vi "Action.vi"(7 "Assert Message":T1, 8 "error in (no error)":errorcluster, 11 "Fail Action Base in":refnum<class "Fail Action Base.lvclass">) -> (0 "error out":errorcluster)   [LabVIEW 2016, in "Assert API Components.lvlib" / "Log Assert Core.lvlib" / "Fail Action Base.lvclass"]
doc: "Dynamic dispatch vi which is triggered when an assert fails and the failure action is set to None. Does nothing"
uses:
  Fail Action Base.lvclass
  Message Data.ctl
  Failure Actions.ctl
  Assert API Components.lvlib
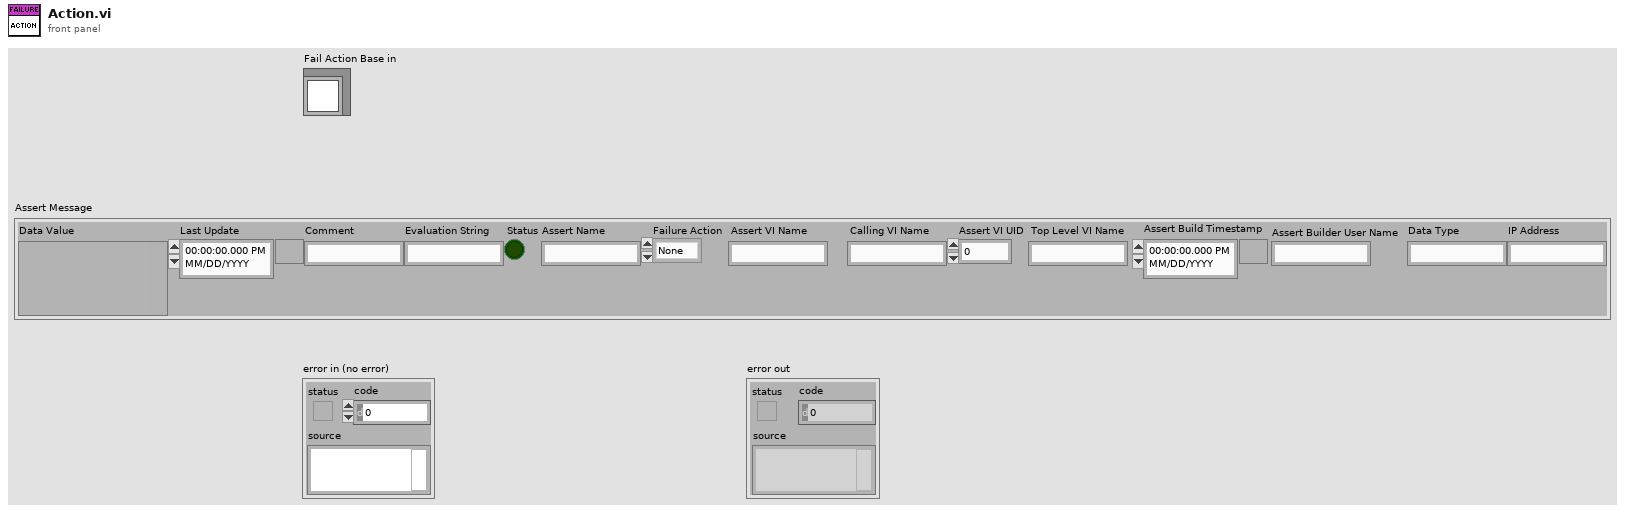
[diagram p1: front panel]
types:
  T1 = typedef "Assert API Components.lvlib/Message Data.ctl" = cluster{"Data Value":variant, "Last Update":timestamp, "Comment":string, "Evaluation String":string, "Status":bool, "Assert Name":string, "Failure Action":T2, "Assert VI Name":string, "Calling VI Name":string, "Assert VI UID":i32, "Top Level VI Name":string, "Assert Build Timestamp":timestamp, "Assert Builder User Name":string, "Data Type":string, "IP Address":string}
  T2 = typedef "Assert API Components.lvlib/Failure Actions.ctl" = enum16{"None", "Log To File", "Pause Execution", "Abort Execution"}
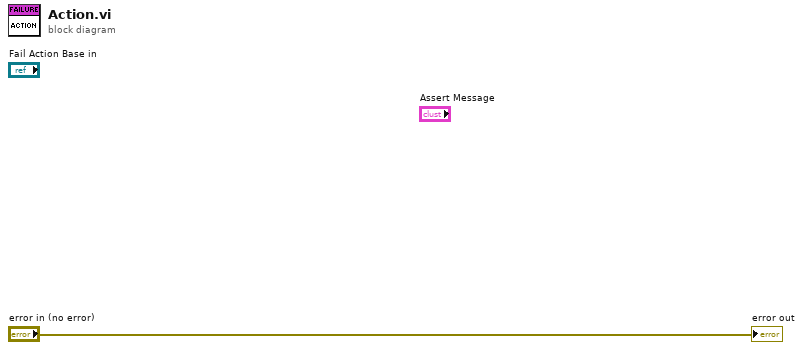
[diagram p0: block diagram]
diagram:
  "error out" <- "error in (no error)"
